vi "Factorial_Calculation.vi"(0 "n":i64) -> (4 "Factorial_of_n":i64, 8 "Sum_of_Factorials_of_First_n_Numbers":i64)   [LabVIEW 2021]
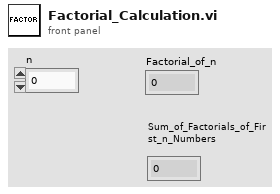
[diagram p1: front panel]
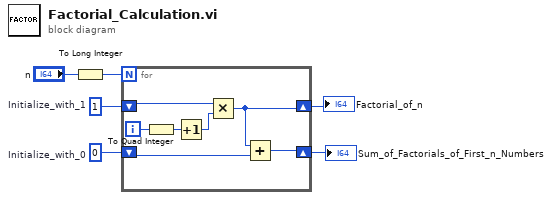
[diagram p0: block diagram]
diagram:
  w5 = i64 0  # Initialize_with_0
  w6 = i64 1  # Initialize_with_1
  n1 = To Long Integer(number="n") -> (32bit integer=w1:i32)
  n2 = for {
    N: w1 -> [_]
    shift-right: [w11] -> w3
    shift-left: w6 -> [w13]
    shift-right: [w10] -> w2
    shift-left: w5 -> [w9]
    i -> [w12]
    n3 = To Quad Integer(1:w12) -> (0:w7:i64)
    n4 = Increment(x=w7) -> (x+1=w8:i64)
    n5 = Multiply(x=w13, y=w8) -> (x*y=w11:i64)
    n6 = Add(x=w11, y=w9) -> (x+y=w10:i64)
  }
  "Factorial_of_n" <- w3
  "Sum_of_Factorials_of_First_n_Numbers" <- w2
